vi "Add Initialization Block Diagram Content.vi"(8 "error in (no error)":errorcluster, 10 "Init":T1, 11 "EST Knock Sensor in":refnum<class "EST Knock Sensor.lvclass">) -> (0 "error out":errorcluster, 3 "EST Knock Sensor out":refnum<class "EST Knock Sensor.lvclass">)   [LabVIEW 2015, in "EST Knock Sensor.lvclass"]
uses:
  EST Knock Sensor.lvclass
  Loop/Block Diagram/Init.Refs.ctl
  <vilib>/Utility/miscctls.llb/LVPointTypeDef.ctl
  Loop/Block Diagram/Block Diagram.lvclass
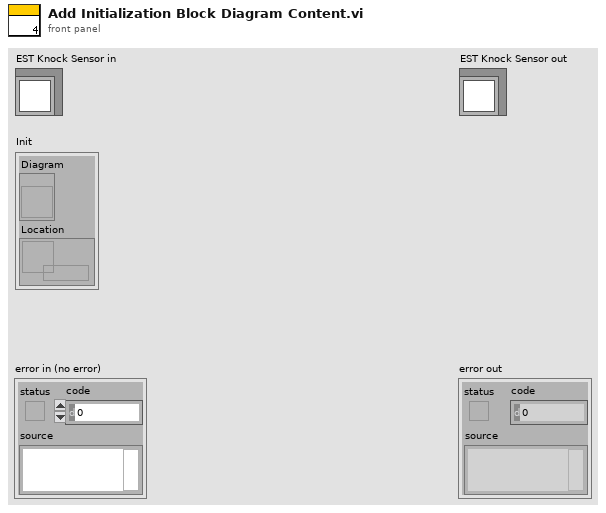
[diagram p1: front panel]
types:
  T1 = typedef "Block Diagram.lvclass/Init.Refs.ctl" = cluster{"Diagram":refnum<vi>, "Location":refnum<data-value>}
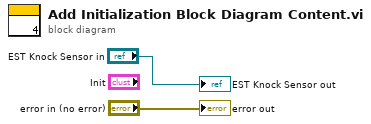
[diagram p0: block diagram]
diagram:
  "error out" <- "error in (no error)"
  "EST Knock Sensor out" <- "EST Knock Sensor in"
